vi "Write VISA.vi"(8 "error in (no error)":errorcluster, 10 "VISA 1":refnum<visa-resource-name>, 11 "MFC in":refnum<class "Scale.lvclass">) -> (0 "error out":errorcluster, 3 "MFC out":refnum<class "Scale.lvclass">)   [LabVIEW 2013, in "Scale.lvlib" / "Scale.lvclass"]
uses:
  Scale.lvclass
  Scale.lvclass/Scale.ctl
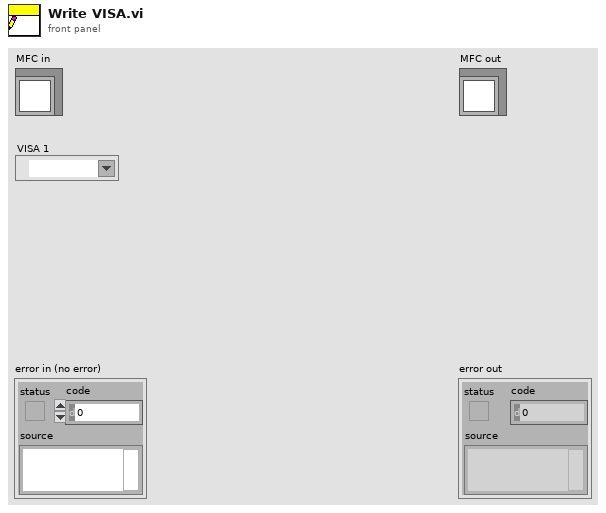
[diagram p1: front panel]
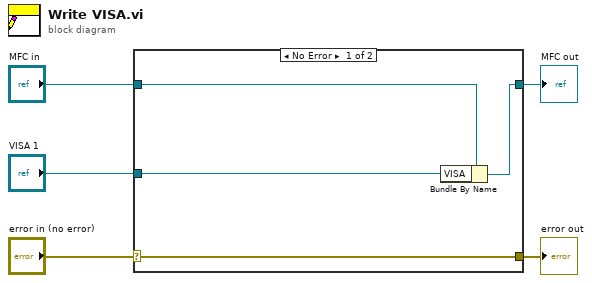
[diagram p0: block diagram]
diagram:
  n1 = case shown="No Error" "error in (no error)" {
    selector: "error in (no error)" -> [w9 w10]
    tunnel: [w9 w10] -> w4
    tunnel: [w7 w11] -> w2
    tunnel: "MFC in" -> [w8 w11]
    tunnel: "VISA 1" -> [w6 _]
    frame No Error {
      n2 = Bundle By Name(cluster=w8, "VISA"=w6) -> (w7:refnum<class "Scale.lvclass">)
    }
    frame Error {
    }
  }
  "error out" <- w4
  "MFC out" <- w2
